vi "IntegerDataTypes.vi"() -> ()   [LabVIEW 2019]
panel:
  in  "U64":u64
  in  "I64":i64
  in  "U32":u32
  in  "I32":i32
  in  "U16":u16
  in  "I16":i16
  in  "U8":u8
  in  "I8":i8
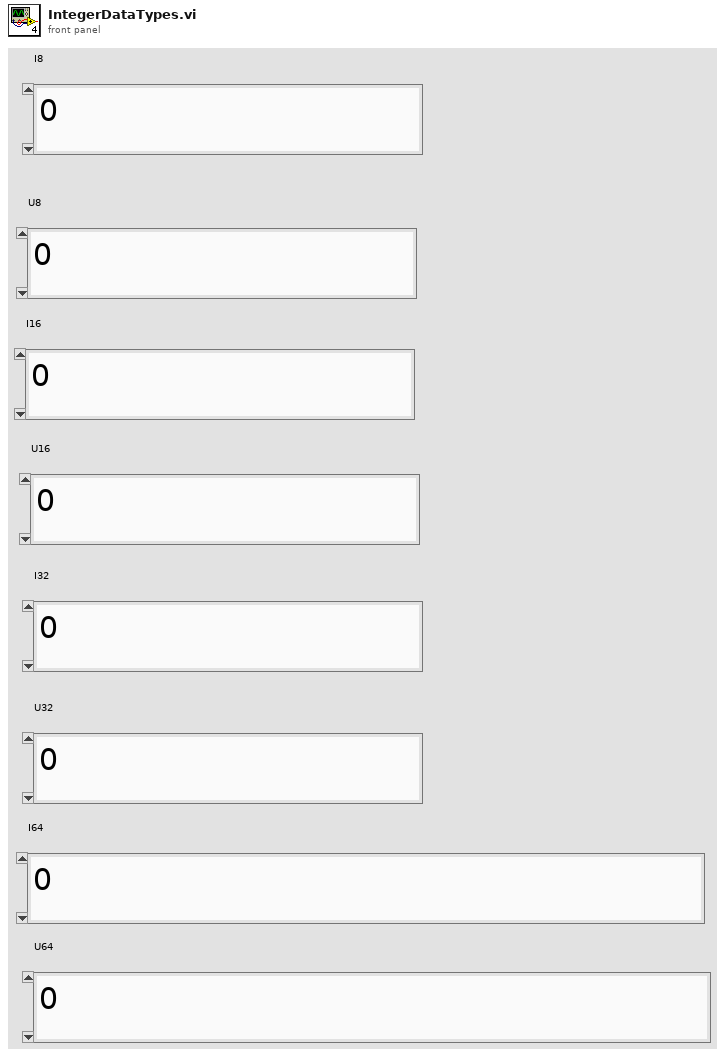
[diagram p1: front panel]
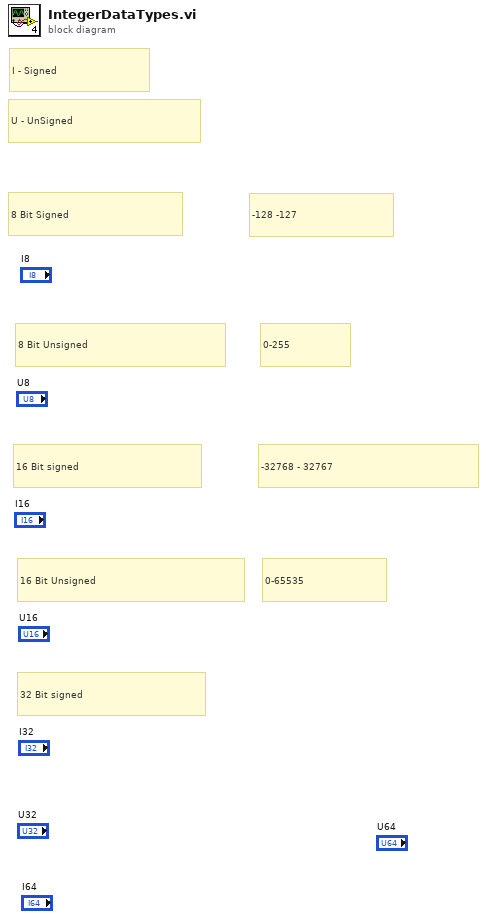
[diagram p0: block diagram]
diagram:
  # "32 Bit signed"
  # "0-65535"
  # "16 Bit Unsigned"
  # "-32768 - 32767"
  # "16 Bit signed"
  # "0-255"
  # "8 Bit Unsigned"
  # "-128 -127"
  # "U - UnSigned"
  # "I - Signed"
  # "8 Bit Signed"
